vi "MeasureSystemTime.vi"(8 "error in":errorcluster, 11 "VISA resource name":refnum<visa-resource-name>) -> (0 "error out":errorcluster, 1 "System time end / us":u32=437417, 2 "System time start / us":u32=437417, 3 "VISA resource name out":refnum<visa-resource-name>)   [LabVIEW 2018, in "GP22_TDC_Arduinoed.lvlib"]
doc: "Gets the system time at the start and end of comms. For use in clock sync via NTP-style algorithm."
uses:
  GP22_TDC_Arduinoed.lvlib
  <vilib>/regexp/Match Regular Expression.xnode
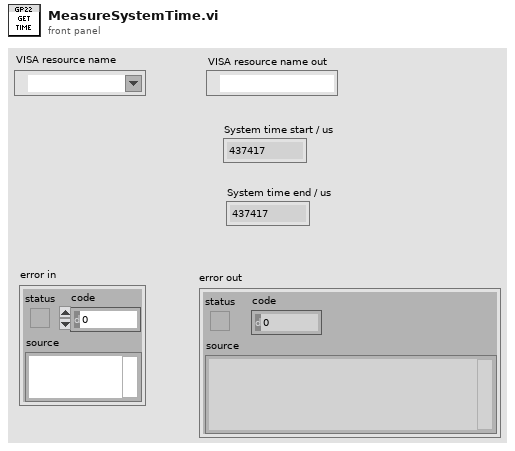
[diagram p1: front panel]
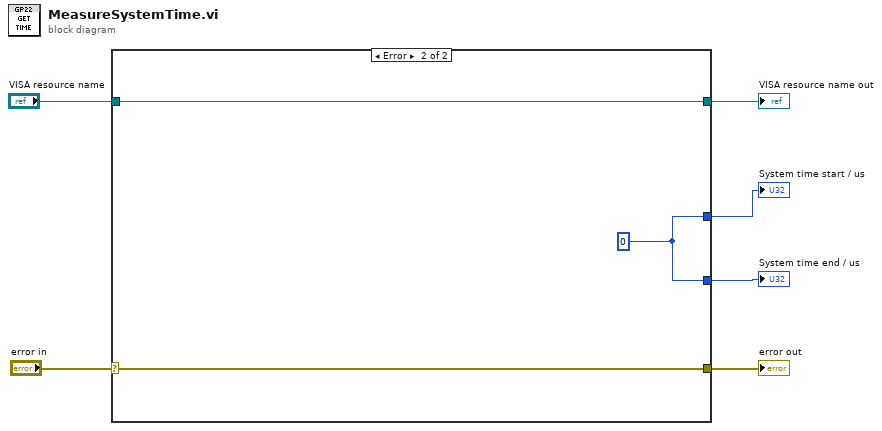
[diagram p0: block diagram]
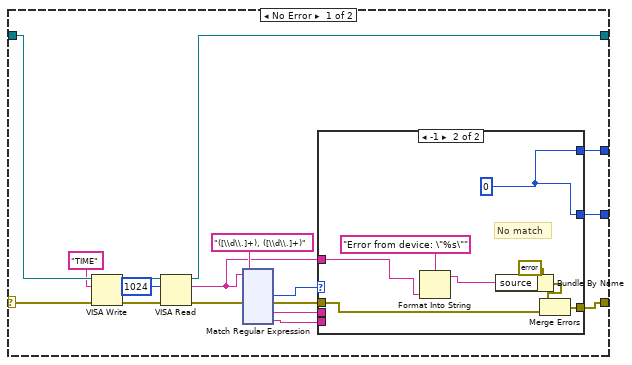
[diagram p2: hidden frame]
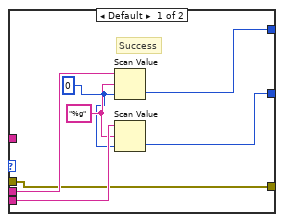
[diagram p3: hidden frame]
diagram:
  n1 = case shown="Error" "error in" {
    selector: "error in" -> [w23 w158]
    tunnel: [w11 w158] -> w5
    tunnel: [w16 w157] -> w4
    tunnel: "VISA resource name" -> [w22 w157]
    tunnel: [w8 w156] -> w2
    tunnel: [w7 w156] -> w1
    frame No Error {
      n2 = VISA Write(VISA resource name=w22, write buffer="TIME", error in (no error)=w23) -> (VISA resource name out=w19:refnum<visa-resource-name>, error out=w20:errorcluster)  [unwired: 1 out]
      n3 = VISA Read(VISA resource name=w19, byte count=u32 1024, error in (no error)=w20) -> (VISA resource name out=w16:refnum<visa-resource-name>, read buffer=w12:string, error out=w17:errorcluster)  [unwired: 1 out]
      n4 = xnode "Match Regular Expression"("input string"=w12, "regular expression"="([\\d\\.]+), ([\\d\\.]+)", "error in"=w17) -> ("offset past match"=w14:i32, "error out"=w13:errorcluster, "submatch 1"=w10:string, "submatch 2"=w9:string)  [unwired: 3 in, 3 out]
      n5 = case shown="-1" w14 {
        tunnel: w13 -> [w28 w35]
        tunnel: w12 -> [_ w34]
        tunnel: [w28 w37] -> w11
        tunnel: w10 -> [w30 _]
        tunnel: w9 -> [w29 _]
        tunnel: [w26 w31] -> w8
        tunnel: [w25 w31] -> w7
        frame Default {
          w24 = u32 0 ("System time end / us")
          w27 = "%g"
          # "Success"
          n6 = Scan Value(string=w30, format string=w27, default (0 dbl)=w24) -> (value=w26:u32)  [unwired: 1 out]
          n7 = Scan Value(string=w29, format string=w27, default (0 dbl)=w24) -> (value=w25:u32)  [unwired: 1 out]
        }
        frame -1 {
          w31 = u32 0
          # "No match"
          n8 = Format Into String(format string="Error from device: \"%s\"", w34) -> (resulting string=w32:string)  [unwired: 2 in, 1 out]
          n9 = Bundle By Name(cluster=errorcluster {"status"=TRUE, "code"=5000, "source"=""} ("error constant"), "source"=w32) -> (w36:errorcluster)
          n10 = Merge Errors(w36, w35) -> (w37:errorcluster)
        }
      }
    }
    frame Error {
      w156 = u32 0
    }
  }
  "VISA resource name out" <- w4
  "error out" <- w5
  "System time start / us" <- w2
  "System time end / us" <- w1
